vi "DecayAnalyzer.vi"() -> ()   [LabVIEW 2014]
uses:
  <vilib>/Analysis/baseanly.llb/Mean (DBL).vi
  <vilib>/gmath/SpecialFunctions.llb/Factorial.vi
  <vilib>/Utility/file.llb/Read From Spreadsheet File (DBL).vi
  <vilib>/imath/engines/lvmath2/RunTimeEngine/Managers/WorkSpace/UID Generator.vi
  <vilib>/imath/engines/lvmath2/RunTimeEngine/RunTimeType/NIMS_RunTimeType_From StrictType (excl LVString).vi
  <instcachedir>/0/NIMS_RunTimeType_From StrictType (excl LVString)_15A5391EEA9C4AACB9955AC755B83D29.lvgen/NIMS_RunTimeType_From StrictType (excl LVString)_15A5391EEA9C4AACB9955AC755B83D29_000.vi
  <vilib>/imath/engines/lvmath2/RunTimeEngine/LocalVariableDefStatement/MC_LocalVariableDefStatement_Display.vi
  <vilib>/imath/engines/lvmath2/RunTimeEngine/Managers/SymbolTable/Clear UID.vi
  <vilib>/imath/engines/lvmath2/RunTimeEngine/NodeEndStatement/NIMS_NodeEndStatement_Output.vi
  <instcachedir>/0/NIMS_NodeEndStatement_Output_53EC0D466D134D7ABD903AC30B43404B.lvgen/NIMS_NodeEndStatement_Output_53EC0D466D134D7ABD903AC30B43404B_004.vi
  <instcachedir>/0/NIMS_NodeEndStatement_Output_53EC0D466D134D7ABD903AC30B43404B.lvgen/NIMS_NodeEndStatement_Output_53EC0D466D134D7ABD903AC30B43404B_005.vi
  <vilib>/imath/engines/lvmath2/RunTimeEngine/ErrorHandling/NIMS_Finalize Error.vi
  <vilib>/Analysis/NI_AALBase.lvlib
  <vilib>/gmath/NI_Gmath.lvlib
  <vilib>/imath/engines/lvmath2/RunTimeEngine/Managers/SymbolTable/NIMS_WorkSpace.lvlib
panel:
  in  "file path (dialog if empty) 2":path=path "C:/Users/eclifton/Documents/GitHub/week8/Constant Rate Data.txt"
  out "Decay Time":dbl=138.56491240254283
  out "Constant Rate":cluster{"X Values":dbl[], "y":dbl[]}[](graph)=[{"X Values"=[5.3125, 15.9375, 26.5625, 37.1875, 47.8125, 58.4375, 69.0625, 79.6875], "y"=[1.0, 0.0, 0.0, 0.0, 1.0, 22.0, 66.0, 31.0]}, {"X Values"=[0.0, 1.0, 2.0, 3.0, 4.0, 5.0, 6.0, 7.0, 8.0, 9.0, 10.0, 11.0, 12.0, 13.0, 14.0, 15.0, 16.0, 17.0, 18.0, 19.0, 20.0, 21.0, 22.0, 23.0, 24.0, 25.0, 26.0, 27.0, 28.0, 29.0, 30.0, 31.0, 32.0, 33.0, 34.0, 35.0, 36.0, 37.0, 38.0, 39.0, 40.0, 41.0, 42.0, 43.0, 44.0, 45.0, 46.0, 47.0, 48.0, 49.0, 50.0, 51.0, 52.0, 53.0, 54.0, 55.0, 56.0, 57.0, 58.0, 59.0, 60.0, 61.0, 62.0, 63.0, 64.0, 65.0, 66.0, 67.0, 68.0, 69.0, 70.0, 71.0, 72.0, 73.0, 74.0, 75.0, 76.0, 77.0, 78.0, 79.0, 80.0, 81.0, 82.0, 83.0, 84.0, 85.0, 86.0, 87.0, 88.0, 89.0], "y"=[9.367734422519673e-28, 6.50863994133247e-26, 2.261079999453805e-24, 5.236611447770838e-23, 9.095907529216824e-22, 1.2639552826136505e-20, 1.463646289384705e-19, 1.4527596640917614e-18, 1.261709761985479e-17, 9.740306674942079e-17, 6.767500679027938e-16, 4.274558843620426e-15, 2.4749460191678323e-14, 1.3227508698756495e-13, 6.564561135209319e-13, 3.0406757831242286e-12, 1.3204008940457329e-11, 5.396504772115935e-11, 2.0830310201643097e-10, 7.617243056338128e-10, 2.646205056803084e-09, 8.755075132838854e-09, 2.764985598864622e-08, 8.352581361715731e-08, 2.418049294350694e-07, 6.72017865044836e-07, 1.7958214213070364e-06, 4.621203149350553e-06, 1.14670764098554e-05, 2.7473271979952794e-05, 6.362749243401188e-05, 0.00014260632601779204, 0.0003096310389544364, 0.0006519078749035681, 0.0013321802392596736, 0.0026445429212411035, 0.005103919269713949, 0.009584241523449893, 0.017523862220018106, 0.03121913746210897, 0.05422712575288226, 0.09189426450402764, 0.1520179224095554, 0.24563034282089793, 0.38786895043112124, 0.5988639607482895, 0.9045363489060133, 1.3371614357750754, 1.9355227600828269, 2.7444661568588846, 3.8136738811095277, 5.1955203886708485, 6.9419484913470795, 9.100414933222345, 11.709089125130129, 14.791632197591131, 18.352014741019577, 22.369927204255706, 26.797375036502952, 31.557015258702947, 36.54267593387268, 41.62231087604222, 46.643397432003056, 51.440514523265094, 55.84457716904568, 59.69298922570464, 62.83983977216362, 65.16523164728999, 66.58290015298574, 67.04544754894613, 66.54676240188786, 65.12147963132013, 62.84162985083888, 59.81088895686658, 56.15704081532024, 52.023387563019, 47.55987595066339, 42.91465891566247, 38.22669395041051, 33.61981546616813, 29.19853188265243, 25.04561346163238, 21.221373954035823, 17.76442206826438, 14.693575002744849, 12.010586781533876, 9.703344519734319, 7.7492179516867505, 6.118301589014888, 4.776354485917742]}]
  in  "file path (dialog if empty)":path=path "C:/Users/eclifton/Documents/GitHub/week8/Decay Data.txt"
  out "Decay Plot":cluster{dbl[], dbl[]}[](graph)=[{[0.0, 0.0, 1.0, 2.0, 3.0, 4.0, 5.0, 6.0, 7.0, 8.0, 9.0, 10.0, 11.0, 12.0, 13.0, 14.0, 15.0, 16.0, 17.0, 18.0, 19.0, 20.0, 21.0, 22.0, 23.0, 24.0, 25.0, 26.0, 27.0, 28.0, 29.0, 30.0, 31.0, 32.0, 33.0, 34.0, 35.0, 36.0, 37.0, 38.0, 39.0, 40.0, 41.0, 42.0, 43.0, 44.0, 45.0, 46.0, 47.0, 48.0, 49.0, 50.0, 51.0, 52.0, 53.0, 54.0, 55.0, 56.0, 57.0, 58.0, 59.0, 60.0, 61.0, 62.0, 63.0, 64.0, 65.0, 66.0, 67.0, 68.0, 69.0, 70.0, 71.0, 72.0, 73.0, 74.0, 75.0, 76.0, 77.0, 78.0, 79.0, 80.0, 81.0, 82.0, 83.0, 84.0, 85.0, 86.0, 87.0, 88.0, 89.0, 90.0, 91.0, 92.0, 93.0, 94.0, 95.0, 96.0, 97.0, 98.0, 99.0, 100.0, 101.0, 102.0, 103.0, 104.0, 105.0, 106.0, 107.0, 108.0, 109.0, 110.0, 111.0, 112.0, 113.0, 114.0, 115.0, 116.0, 117.0, 118.0, 119.0, 120.0, 121.0, 122.0, 123.0, 124.0, 125.0, 126.0, 127.0, 128.0, 129.0, 130.0, 131.0, 132.0, 133.0, 134.0, 135.0, 136.0, 137.0, 138.0, 139.0, 140.0, 141.0, 142.0, 143.0, 144.0, 145.0, 146.0, 147.0, 148.0, 149.0, 150.0, 151.0, 152.0, 153.0, 154.0, 155.0, 156.0, 157.0, 158.0, 159.0, 160.0, 161.0, 162.0, 163.0, 164.0, 165.0, 166.0, 167.0, 168.0, 169.0, 170.0, 171.0, 172.0, 173.0, 174.0, 175.0, 176.0, 177.0, 178.0, 179.0, 180.0, 181.0, 182.0, 183.0, 184.0, 185.0, 186.0, 187.0, 188.0, 189.0, 190.0, 191.0, 192.0, 193.0, 194.0, 195.0, 196.0, 197.0, 198.0, 199.0, 200.0, 201.0, 202.0, 203.0, 204.0, 205.0, 206.0, 207.0, 208.0, 209.0, 210.0, 211.0, 212.0, 213.0, 214.0, 215.0, 216.0, 217.0, 218.0, 219.0, 220.0, 221.0, 222.0, 223.0, 224.0, 225.0, 226.0, 227.0, 228.0, 229.0, 230.0, 231.0, 232.0, 233.0, 234.0, 235.0, 236.0, 237.0, 238.0, 239.0, 240.0, 241.0, 242.0, 243.0, 244.0, 245.0, 246.0, 247.0, 248.0, 249.0, 250.0, 251.0, 252.0, 253.0, 254.0, 255.0, 256.0, 257.0, 258.0, 259.0, 260.0, 261.0, 262.0, 263.0, 264.0, 265.0, 266.0, 267.0, 268.0, 269.0, 270.0, 271.0, 272.0, 273.0, 274.0, 275.0, 276.0, 277.0, 278.0, 279.0, 280.0, 281.0, 282.0, 283.0, 284.0, 285.0, 286.0, 287.0, 288.0, 289.0, 290.0, 291.0, 292.0, 293.0, 294.0, 295.0, 296.0, 297.0, 298.0, 299.0, 300.0], [0.0, 0.0, 75.0, 86.0, 72.0, 76.0, 79.0, 69.0, 66.0, 83.0, 71.0, 77.0, 89.0, 72.0, 85.0, 73.0, 68.0, 70.0, 68.0, 83.0, 74.0, 76.0, 59.0, 63.0, 80.0, 69.0, 62.0, 71.0, 69.0, 59.0, 65.0, 72.0, 59.0, 65.0, 61.0, 71.0, 68.0, 52.0, 67.0, 49.0, 60.0, 73.0, 48.0, 54.0, 58.0, 70.0, 69.0, 68.0, 56.0, 51.0, 69.0, 66.0, 50.0, 50.0, 58.0, 44.0, 58.0, 59.0, 44.0, 44.0, 48.0, 59.0, 61.0, 56.0, 52.0, 60.0, 55.0, 49.0, 43.0, 51.0, 47.0, 53.0, 62.0, 41.0, 40.0, 44.0, 41.0, 46.0, 48.0, 51.0, 48.0, 42.0, 49.0, 43.0, 45.0, 46.0, 48.0, 49.0, 64.0, 39.0, 52.0, 40.0, 42.0, 32.0, 26.0, 42.0, 45.0, 38.0, 46.0, 35.0, 33.0, 27.0, 29.0, 44.0, 40.0, 38.0, 32.0, 37.0, 46.0, 41.0, 31.0, 38.0, 30.0, 24.0, 33.0, 33.0, 23.0, 30.0, 36.0, 31.0, 42.0, 34.0, 32.0, 36.0, 39.0, 26.0, 32.0, 34.0, 28.0, 22.0, 31.0, 41.0, 24.0, 22.0, 28.0, 20.0, 35.0, 30.0, 24.0, 34.0, 27.0, 30.0, 33.0, 26.0, 20.0, 28.0, 30.0, 31.0, 31.0, 19.0, 24.0, 23.0, 24.0, 21.0, 23.0, 22.0, 27.0, 19.0, 29.0, 17.0, 30.0, 30.0, 31.0, 28.0, 24.0, 24.0, 21.0, 25.0, 21.0, 22.0, 18.0, 19.0, 26.0, 21.0, 19.0, 24.0, 20.0, 17.0, 19.0, 19.0, 14.0, 23.0, 19.0, 20.0, 20.0, 16.0, 15.0, 13.0, 15.0, 17.0, 14.0, 15.0, 23.0, 14.0, 20.0, 22.0, 23.0, 14.0, 14.0, 19.0, 13.0, 14.0, 17.0, 9.0, 16.0, 13.0, 17.0, 16.0, 15.0, 17.0, 17.0, 14.0, 15.0, 12.0, 9.0, 12.0, 14.0, 21.0, 24.0, 16.0, 14.0, 13.0, 18.0, 23.0, 13.0, 7.0, 14.0, 10.0, 14.0, 13.0, 19.0, 8.0, 14.0, 15.0, 8.0, 15.0, 12.0, 10.0, 12.0, 11.0, 9.0, 17.0, 10.0, 8.0, 15.0, 14.0, 11.0, 10.0, 16.0, 12.0, 18.0, 12.0, 12.0, 19.0, 11.0, 8.0, 20.0, 16.0, 15.0, 9.0, 12.0, 7.0, 9.0, 9.0, 9.0, 8.0, 16.0, 8.0, 12.0, 12.0, 16.0, 7.0, 14.0, 10.0, 12.0, 13.0, 11.0, 4.0, 10.0, 13.0, 10.0, 8.0, 11.0, 19.0, 13.0, 11.0, 12.0, 10.0, 6.0, 6.0, 7.0, 8.0, 7.0, 8.0, 13.0, 10.0, 8.0, 18.0, 5.0, 10.0, 12.0, 13.0]}, {[0.0, 0.0, 1.0, 2.0, 3.0, 4.0, 5.0, 6.0, 7.0, 8.0, 9.0, 10.0, 11.0, 12.0, 13.0, 14.0, 15.0, 16.0, 17.0, 18.0, 19.0, 20.0, 21.0, 22.0, 23.0, 24.0, 25.0, 26.0, 27.0, 28.0, 29.0, 30.0, 31.0, 32.0, 33.0, 34.0, 35.0, 36.0, 37.0, 38.0, 39.0, 40.0, 41.0, 42.0, 43.0, 44.0, 45.0, 46.0, 47.0, 48.0, 49.0, 50.0, 51.0, 52.0, 53.0, 54.0, 55.0, 56.0, 57.0, 58.0, 59.0, 60.0, 61.0, 62.0, 63.0, 64.0, 65.0, 66.0, 67.0, 68.0, 69.0, 70.0, 71.0, 72.0, 73.0, 74.0, 75.0, 76.0, 77.0, 78.0, 79.0, 80.0, 81.0, 82.0, 83.0, 84.0, 85.0, 86.0, 87.0, 88.0, 89.0, 90.0, 91.0, 92.0, 93.0, 94.0, 95.0, 96.0, 97.0, 98.0, 99.0, 100.0, 101.0, 102.0, 103.0, 104.0, 105.0, 106.0, 107.0, 108.0, 109.0, 110.0, 111.0, 112.0, 113.0, 114.0, 115.0, 116.0, 117.0, 118.0, 119.0, 120.0, 121.0, 122.0, 123.0, 124.0, 125.0, 126.0, 127.0, 128.0, 129.0, 130.0, 131.0, 132.0, 133.0, 134.0, 135.0, 136.0, 137.0, 138.0, 139.0, 140.0, 141.0, 142.0, 143.0, 144.0, 145.0, 146.0, 147.0, 148.0, 149.0, 150.0, 151.0, 152.0, 153.0, 154.0, 155.0, 156.0, 157.0, 158.0, 159.0, 160.0, 161.0, 162.0, 163.0, 164.0, 165.0, 166.0, 167.0, 168.0, 169.0, 170.0, 171.0, 172.0, 173.0, 174.0, 175.0, 176.0, 177.0, 178.0, 179.0, 180.0, 181.0, 182.0, 183.0, 184.0, 185.0, 186.0, 187.0, 188.0, 189.0, 190.0, 191.0, 192.0, 193.0, 194.0, 195.0, 196.0, 197.0, 198.0, 199.0, 200.0, 201.0, 202.0, 203.0, 204.0, 205.0, 206.0, 207.0, 208.0, 209.0, 210.0, 211.0, 212.0, 213.0, 214.0, 215.0, 216.0, 217.0, 218.0, 219.0, 220.0, 221.0, 222.0, 223.0, 224.0, 225.0, 226.0, 227.0, 228.0, 229.0, 230.0, 231.0, 232.0, 233.0, 234.0, 235.0, 236.0, 237.0, 238.0, 239.0, 240.0, 241.0, 242.0, 243.0, 244.0, 245.0, 246.0, 247.0, 248.0, 249.0, 250.0, 251.0, 252.0, 253.0, 254.0, 255.0, 256.0, 257.0, 258.0, 259.0, 260.0, 261.0, 262.0, 263.0, 264.0, 265.0, 266.0, 267.0, 268.0, 269.0, 270.0, 271.0, 272.0, 273.0, 274.0, 275.0, 276.0, 277.0, 278.0, 279.0, 280.0, 281.0, 282.0, 283.0, 284.0, 285.0, 286.0, 287.0, 288.0, 289.0, 290.0, 291.0, 292.0, 293.0, 294.0, 295.0, 296.0, 297.0, 298.0, 299.0, 300.0], [77.39664797388384, 77.39664797388384, 76.84009987035847, 76.28755382376508, 75.73898105589105, 75.19435299546362, 74.65364127666197, 74.11681773763985, 73.58385441905868, 73.0547235626315, 72.52939760967713, 72.00784919968496, 71.49005116888975, 70.97597654885706, 70.46559856507852, 69.95889063557739, 69.45582636952405, 68.95637956586157, 68.46052421194099, 67.96823448216657, 67.47948473665069, 66.99424951987844, 66.51250355938186, 66.03422176442363, 65.55937922469032, 65.08795120899494, 64.61991316398887, 64.15524071288314, 63.693909654178654, 63.23589596040588, 62.78117577687328, 62.32972542042499, 61.881521378207296, 61.43654030644398, 60.99475902922059, 60.55615453727729, 60.1207039868105, 59.688384698283166, 59.25917415524347, 58.83305000315216, 58.409990048218226, 57.98997225624303, 57.57297475147264, 57.15897581545853, 56.74795388592638, 56.33988755565308, 55.93475557135174, 55.5325368325648, 55.13321039056506, 54.73675544726457, 54.3431513541314, 53.95237761111426, 53.56441386557475, 53.179239911227356, 52.79683568708703, 52.41718127642438, 52.04025690572833, 51.66604294367625, 51.29451990011154, 50.925668425028476, 50.55946930756443, 50.19590347499931, 49.83495199176219, 49.47659605844513, 49.12081701082396, 48.7675963188863, 48.416915585866356, 48.068756547286874, 47.72310107000777, 47.37993115128177, 47.039228917816736, 46.700976624844806, 46.365156655198184, 46.03175151839155, 45.700743849711145, 45.372116409310394, 45.045852081311914, 44.72193387291614, 44.40034491351627, 44.08106845381961, 43.764087864975195, 43.44938663770772, 43.13694838145769, 42.826756823527774, 42.51879580823523, 42.2130492960705, 41.90950136286183, 41.60813619894587, 41.30893810834429, 41.011891507946245, 40.716980926696806, 40.42419100479117, 40.13350649287464, 39.84491225124843, 39.55839324908117, 39.273934563626014, 38.99152137944339, 38.71113898762946, 38.432772785049956, 38.15640827357965, 37.88203105934724, 37.60962685198566, 37.339181463887805, 37.07068080946761, 36.80411090442644, 36.53945786502467, 36.27670790735872, 36.01584734664299, 35.756862596497264, 35.49974016823896, 35.24446667018069, 34.991028806932775, 34.73941337871072, 34.489607280647796, 34.24159750211247, 33.995371126030776, 33.75091532821356, 33.50821737668856, 33.26726463103729, 33.028044541736676, 32.790544649505456, 32.55475258465525, 32.320656066446325, 32.08824290244797, 31.857500987903496, 31.628418305099736, 31.40098292274118, 31.17518299532854, 30.951006762541805, 30.7284425486277, 30.50747876179163, 30.288103893593917, 30.07030651835038, 29.854075292537328, 29.639398954200658, 29.42626632236938, 29.21466629647325, 29.004587855764612, 28.79602005874441, 28.58895204259233, 28.383373022601024, 28.179272291614428, 27.976639219470073, 27.77546325244546, 27.57573391270838, 27.377440797771186, 27.180573579949048, 26.985122005822, 26.79107589570094, 26.598425143097437, 26.407159714197366, 26.21726964733831, 26.02874505249069, 25.841576110742757, 25.655753073789093, 25.471266263422955, 25.288106071032175, 25.10626295709873, 24.92572745070189, 24.74649014902496, 24.56854171686551, 24.39187288614923, 24.216474455447173, 24.042337289496555, 23.869452318724928, 23.697810538777834, 23.52740301004983, 23.358220857218893, 23.19025526878412, 23.02349749660688, 22.85793885545511, 22.693570722551016, 22.53038453712194, 22.368371799954517, 22.20752407295197, 22.047832978694686, 21.889290200003835, 21.73188747950825, 21.57561661921429, 21.420469480078932, 21.26643798158582, 21.113514101324423, 20.961689874572205, 20.810957393879804, 20.661308808659168, 20.5127363247747, 20.365232204137307, 20.21878876430137, 20.07339837806463, 19.929053473070923, 19.785746531415825, 19.643470089255064, 19.502216736415786, 19.361979116010627, 19.22274992405454, 19.084521909084366, 18.94728787178118, 18.811040664595314, 18.675773191374095, 18.541478406992265, 18.40814931698503, 18.275778977183787, 18.14436049335445, 18.01388702083837, 17.88435176419585, 17.755747976852206, 17.628068960746415, 17.501308065982236, 17.375458690481857, 17.25051427964207, 17.126468325992864, 17.003314368858504, 16.88104599402104, 16.759656833386234, 16.6391405646519, 16.519490910978607, 16.400701640662763, 16.282766566812064, 16.165679547023252, 16.049434483062207, 15.934025320546315, 15.819446048629166, 15.705690699687471, 15.59275334901026, 15.4806281144903, 15.369309156317737, 15.258790676675954, 15.14906691943959, 15.040132169874749, 14.93198075434136, 14.82460703999768, 14.718005434506916, 14.612170385745953, 14.507096381516199, 14.402777949256482, 14.299209655758027, 14.196386106881473, 14.094301947275945, 13.992951860100108, 13.892330566745283, 13.792432826560479, 13.693253436579484, 13.594787231249866, 13.497029082163921, 13.399973897791597, 13.303616623215287, 13.20795223986657, 13.112975765264832, 13.01868225275774, 12.925066791263633, 12.832124505015734, 12.73985055330819, 12.64824013024396, 12.557288464484534, 12.466990819001381, 12.37734249082928, 12.288338810821333, 12.199975143405819, 12.112246886344732, 12.0251494704941, 11.938678359566, 11.852829049892305, 11.767597070190108, 11.682977981328856, 11.598967376099141, 11.515560878983154, 11.432754145926811, 11.35054286411349, 11.268922751739403, 11.187889557790605, 11.10743906182157, 11.027567073735387, 10.948269433565528, 10.869542011259181, 10.791380706462142, 10.713781448305271, 10.636740195192452, 10.560252934590103, 10.484315682818197, 10.408924484842766, 10.33407541406992, 10.259764572141345, 10.185988088731252, 10.112742121344802, 10.040022855117996, 9.967826502618944, 9.896149303650658, 9.824987525055166, 9.7543374605191, 9.684195430380658, 9.614557781437952, 9.54542088675874, 9.476781145491524, 9.408634982678011, 9.340978849066916, 9.273809220929104, 9.207122599874069, 9.140915512667725, 9.07518451105151, 9.00992617156279, 8.945137095356563, 8.880813908028408]}]
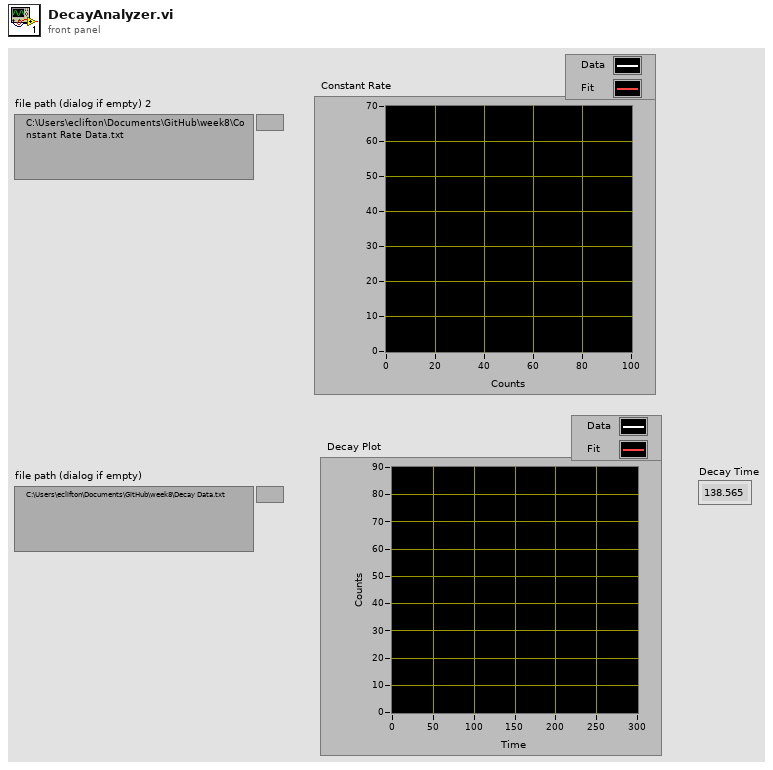
[diagram p1: front panel]
types:
  T1 = cluster{"X Values":dbl[], "Histogram: h(x)":i32[]}
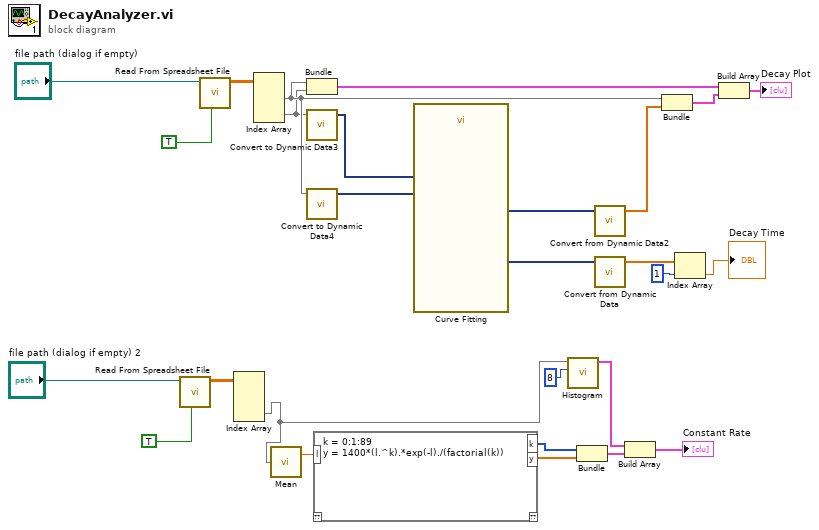
[diagram p0: block diagram]
diagram:
  n1 = call-poly <vilib>:"Read From Spreadsheet File.vi"("transpose (no:F)"=TRUE, "file path (dialog if empty)"="file path (dialog if empty) 2") -> ("all rows"=w4:dbl[][])  [unwired: 5 in, 4 out]
  n2 = call-poly <vilib>:"Read From Spreadsheet File.vi"("transpose (no:F)"=TRUE, "file path (dialog if empty)"="file path (dialog if empty)") -> ("all rows"=w19:dbl[][])  [unwired: 5 in, 4 out]
  n3 = Index Array(array=w4) -> (element #2=w2:dbl[])  [unwired: 4 in, 1 out]
  n4 = Index Array(array=w19) -> (element #1=w14:dbl[], element #2=w9:dbl[])  [unwired: 4 in]
  n5 = call-poly <vilib>:"Mean.vi"("X"=w2) -> ("mean"=w11:dbl)  [unwired: 1 out]
  n6 = Bundle("all rows"=w14, "all rows"=w9) -> (w15:cluster{"all rows":dbl[], "all rows":dbl[]})  [unwired: 1 in]
  n7 = call "Convert to Dynamic Data3"("Array"=w9) -> ("Dynamic Data Type"=w18:dynamicdata)  [unwired: 3 in]
  n8 = call "Convert to Dynamic Data4"("Array"=w14) -> ("Dynamic Data Type"=w17:dynamicdata)  [unwired: 3 in]
  n9 = mathscript code="k = 0:1:89\ny = 1400*(l.^k).*exp(-l)./(factorial(k))"("l"=w11) -> ("y"=w10:dbl[], "k"=w1:i32[])  [unwired: 1 in, 1 out]
  n10 = call "Curve Fitting"("Locations"=w17, "Signals"=w18) -> ("best fit"=w27:dynamicdata, "non-linear coefficients"=w24:dynamicdata)  [unwired: 5 in, 3 out]
  n11 = call <vilib>:"Histogram.vi"("intervals"=8, "X"=w2) -> ("Histogram Graph"=w8:T1)  [unwired: 6 in, 3 out]
  n12 = Bundle("k"=w1, "y"=w10) -> (w3:cluster{"k":i32[], "y":dbl[]})  [unwired: 1 in]
  n13 = call "Convert from Dynamic Data2"("Dynamic Data Type"=w27) -> ("Array"=w25:dbl[])  [unwired: 3 in]
  n14 = call "Convert from Dynamic Data"("Dynamic Data Type"=w24) -> ("Array"=w22:dbl[])  [unwired: 3 in]
  n15 = Build Array(w8, w3) -> (→"Constant Rate":cluster{"X Values":dbl[], "y":dbl[]}[])
  n16 = Bundle("all rows"=w14, "Array"=w25) -> (w26:cluster{"all rows":dbl[], "Array":dbl[]})  [unwired: 1 in]
  n17 = Index Array(array=w22, index=1) -> (element=→"Decay Time":dbl)
  n18 = Build Array(w15, w26) -> (→"Decay Plot":cluster{"all rows":dbl[], "Array":dbl[]}[])
